vi "8HP_Standard_Clone.vi"(0 "Single 8HP":T1) -> (2 "DAQ Error":errorcluster, 3 "All samples out":sgl[][](array[numeric]), 4 "Ch No":i16[](array[numeric]), 5 "Index":i32[](array[numeric]), 6 "Sampling Rate Hz":dbl)   [LabVIEW 2021]
doc: "Use this plug-in with the Nathan 7609 data acquisition system"
uses:
  Device ID port info.ctl
  ctls/8HP_Cmd (USB).ctl
  Globals/Meas_global.vi
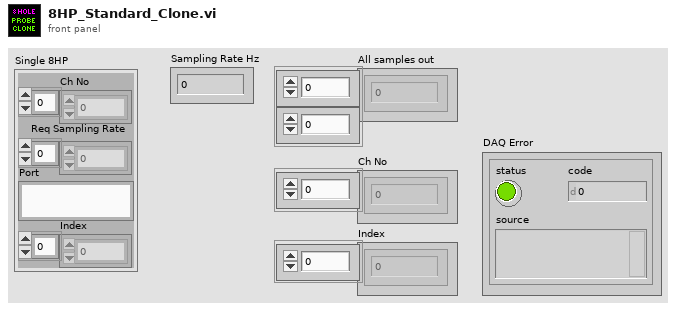
[diagram p1: front panel]
types:
  T1 = typedef "Device ID port info.ctl" = cluster{"Ch No":i16[], "Req Sampling Rate":dbl[], "Port":string, "Index":i32[]}
  T2 = typedef "8HP_Cmd (USB).ctl" = string
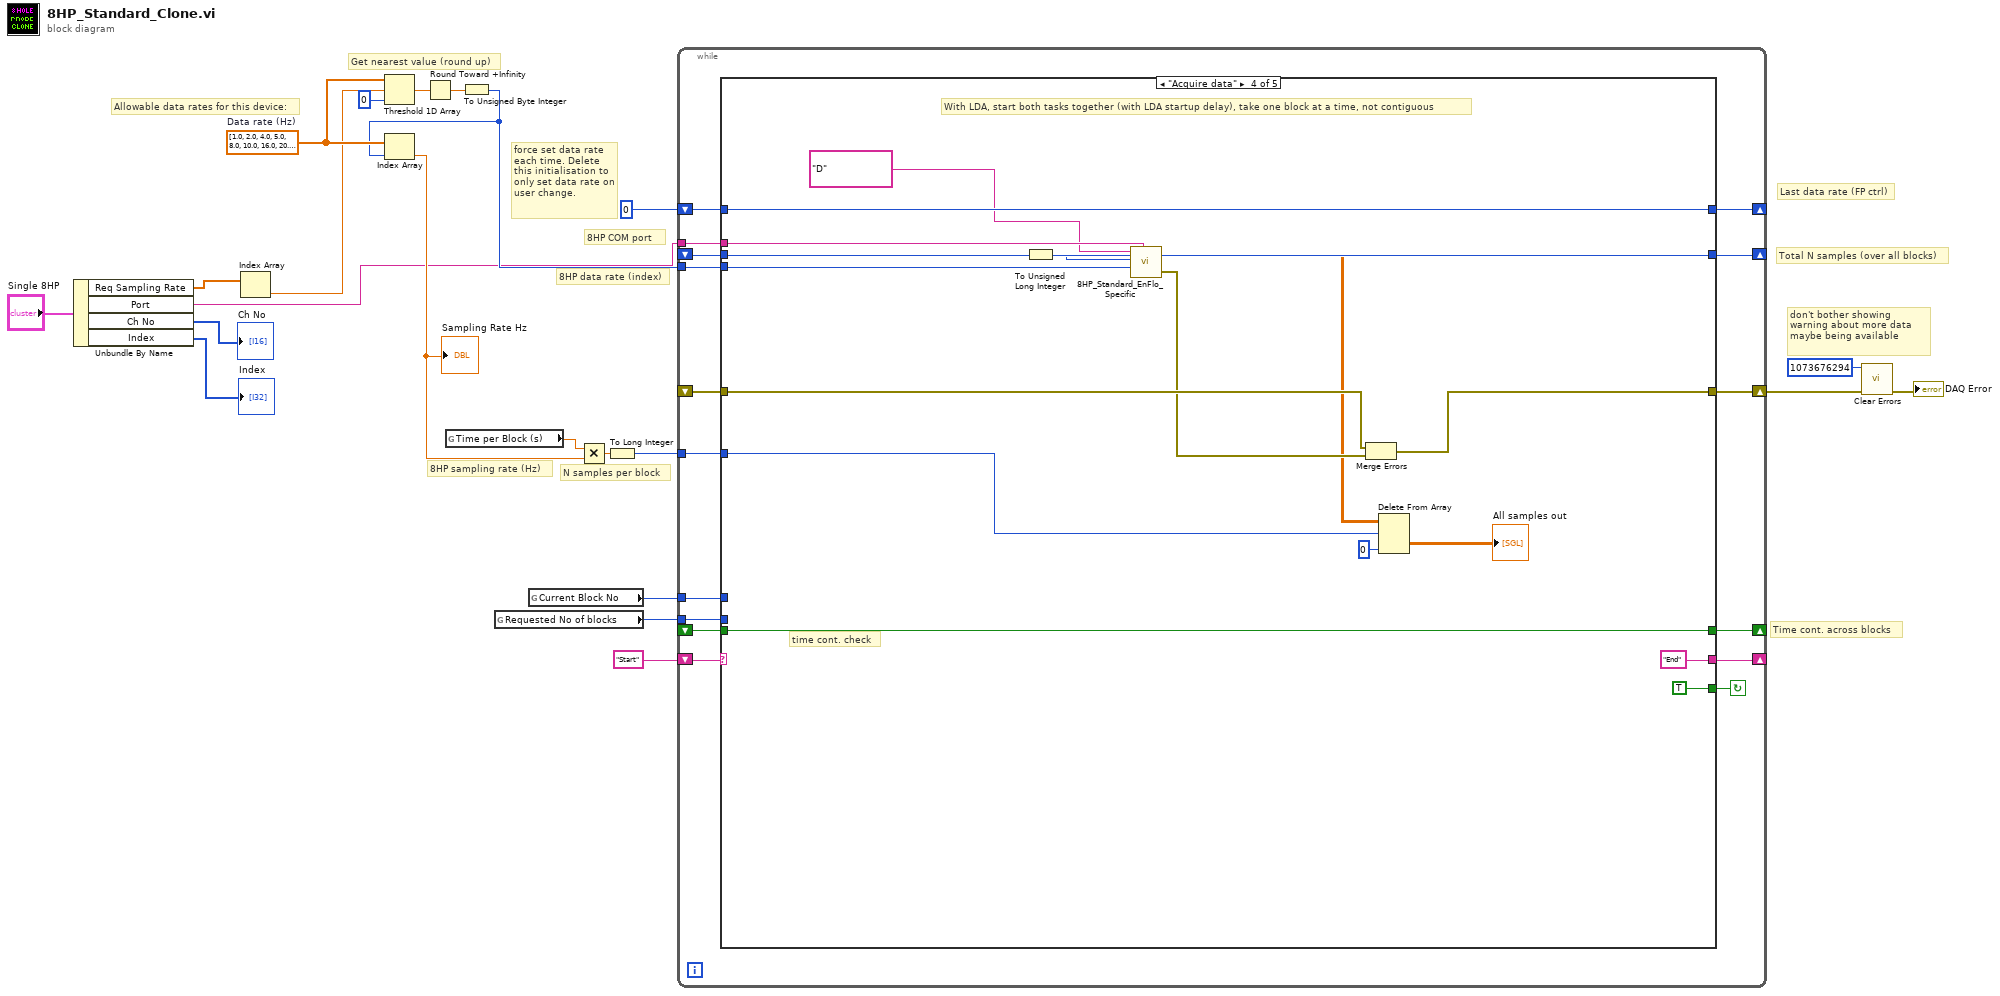
[diagram p0: block diagram]
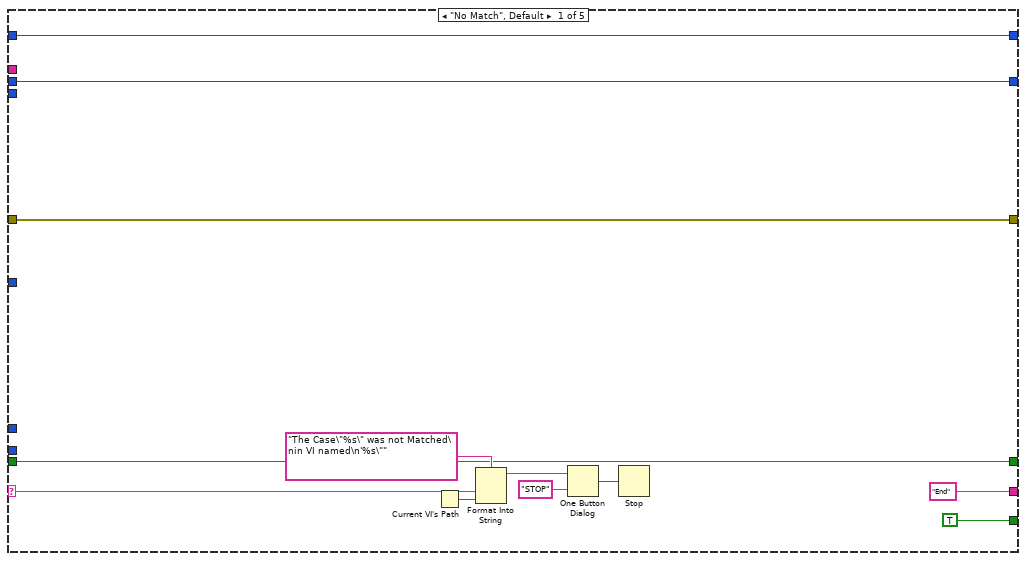
[diagram p2: hidden frame]
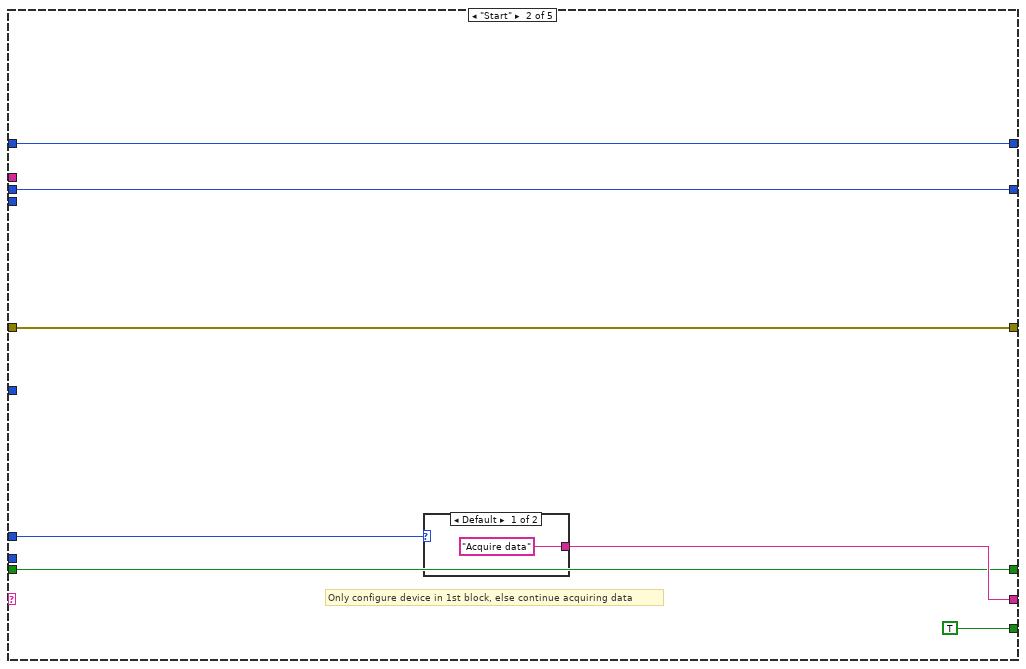
[diagram p3: hidden frame]
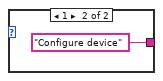
[diagram p4: hidden frame]
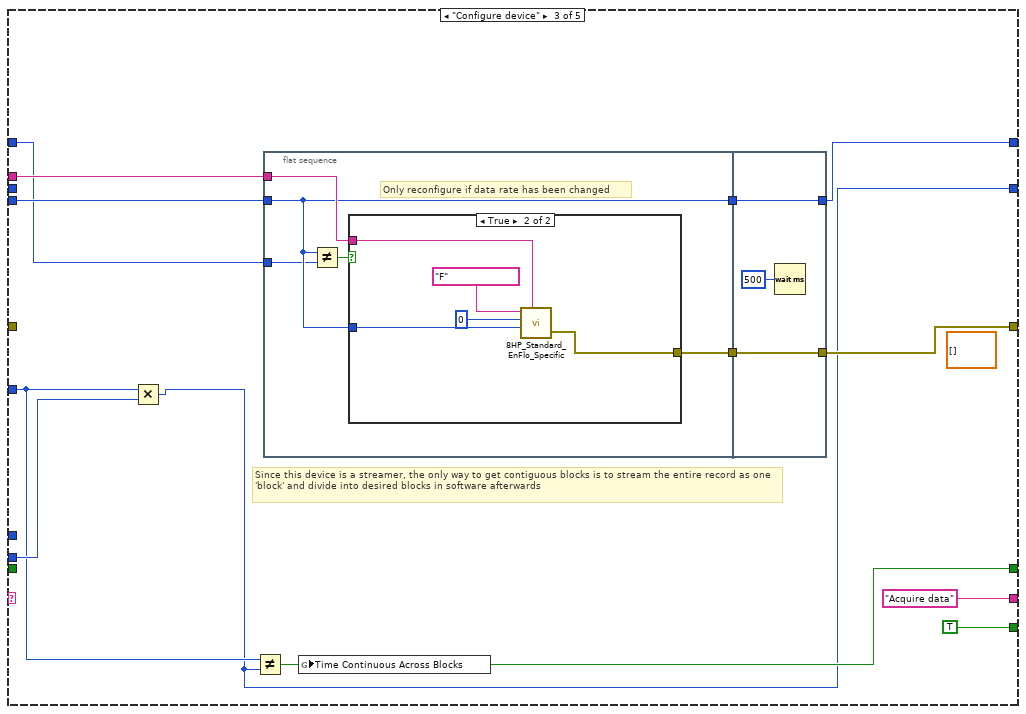
[diagram p5: hidden frame]
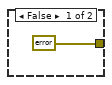
[diagram p6: hidden frame]
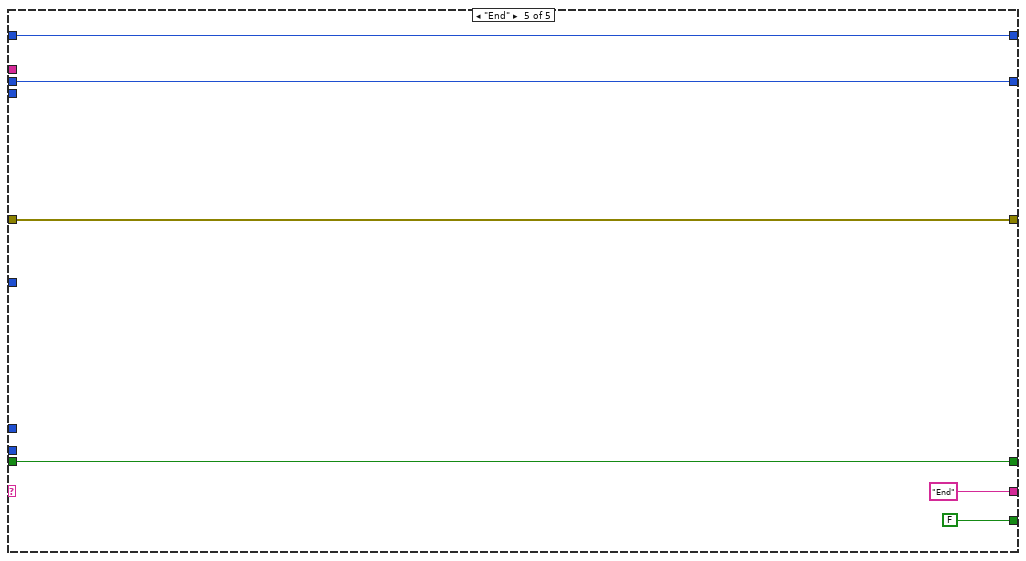
[diagram p7: hidden frame]
diagram:
  w13 = dbl[] [1.0, 2.0, 4.0, 5.0, 8.0, 10.0, 16.0, 20.0, 25.0, 32.0, 40.0, 50.0, 64.0, 80.0, 100.0, 125.0, 160.0, 200.0, 250.0, 320.0, 400.0, 500.0, 625.0, 800.0, 1000.0]  # Data rate (Hz)
  # "N samples per block"
  # "8HP sampling rate (Hz)"
  # "8HP COM port"
  # "8HP data rate (index)"
  # "Allowable data rates for this device:"
  # "Get nearest value (round up)"
  # "force set data rate each time. Delete this initialisation to only set data rate on user change."
  # "Last data rate (FP ctrl)"
  # "Total N samples (over all blocks)"
  # "don't bother showing warning about more data maybe being available"
  # "Time cont. across blocks"
  n1 = Unbundle By Name("Single 8HP") -> ("Req Sampling Rate"=w4:dbl[], "Port"=w5:string, "Ch No"=→"Ch No":i16[], "Index"=→"Index":i32[])
  n2 = Index Array(array=w4) -> (element=w3:dbl)  [unwired: 1 in]
  n3 = Threshold 1D Array(1:0 ("start index (0)"), 2:w3, 3:w13) -> (0:w14:dbl)
  n4 = Round Toward +Infinity(x=w14) -> (ceil(x): smallest int >= x=w12:dbl)
  n5 = global read "Meas_global.vi" "Time per Block (s)"() -> (w11:dbl)
  n6 = To Unsigned Byte Integer(number=w12) -> (unsigned 8bit integer=w7:u8)
  n7 = Index Array(array=w13, index=w7) -> (element=w8:dbl)
  "Sampling Rate Hz" <- w8
  n8 = global read "Meas_global.vi" "Requested No of blocks"() -> (w20:i32)
  n9 = global read "Meas_global.vi" "Current Block No"() -> (w21:i32)
  n10 = Multiply(x=w11, y=w8) -> (x*y=w10:dbl)
  n11 = To Long Integer(number=w10) -> (32bit integer=w9:i32)
  n12 = while {
    shift-left: "Start" -> [w38]
    shift-right: [w31] -> _
    tunnel: w9 -> [w37]
    tunnel: w21 -> [w36]
    tunnel: w20 -> [w34]
    shift-right: [w32] -> w17
    shift-left: _ -> [w33]
    shift-right: [w30] -> _
    shift-left: _ -> [w29]
    tunnel: w5 -> [w28]
    tunnel: w7 -> [w27]
    shift-right: [w26] -> _
    shift-left: _ -> [w25]
    shift-right: [w24] -> _
    shift-left: u8 0 ("Pressure data rate (Hz)") -> [w23]
    stop <- w35 continue-if-true
    n13 = case shown="\"Acquire data\"" w38 {
      selector: w38 -> [w43 _ _ _ _]
      tunnel: ["End" w54 "Acquire data" ("f") "End" "End" ("f")] -> w31
      tunnel: w37 -> [_ _ w68 w97 _]
      tunnel: w36 -> [_ w55 _ _ _]
      tunnel: [TRUE TRUE TRUE TRUE FALSE] -> w35
      tunnel: w34 -> [_ _ w71 _ _]
      tunnel: w33 -> [w42 w56 _ w100 w105]
      tunnel: [w42 w56 w70 w98 w105] -> w32
      tunnel: [w41 w53 w67 w99 w106] -> w30
      tunnel: w29 -> [w41 w53 _ w99 w106]
      tunnel: w28 -> [_ _ w66 w96 _]
      tunnel: w27 -> [_ _ w65 w95 _]
      tunnel: [w39 w51 w62 w93 w103] -> w26
      tunnel: w25 -> [w39 w51 _ w93 w103]
      tunnel: [w40 w52 w64 w94 w104] -> w24
      tunnel: w23 -> [w40 w52 w63 w94 w104]
      frame "No Match", Default {
        n14 = Current VI's Path() -> (path=w46:path)
        n15 = Format Into String(format string="The Case\"%s\" was not Matched\nin VI named\n'%s\"" ("Format String"), w43, w46) -> (resulting string=w49:string)  [unwired: 2 in, 1 out]
        n16 = One Button Dialog(message=w49, button name ("OK")="STOP") -> (true=w47:bool)
        n17 = Stop(stop? (T)=w47) -> ()
      }
      frame "Start" {
        # "Only configure device in 1st block, else continue acquiring data"
        n18 = case shown="Default" w55 {
          tunnel: ["Acquire data" ("f") "Configure device" ("f")] -> w54
          frame Default {
          }
          frame 1 {
          }
        }
      }
      frame "Configure device" {
        (unwired) sgl[][] [] ("Channel volts")
        # "Since this device is a streamer, the only way to get contiguous blocks is to stream the entire record as one 'block' and divide into desired blocks in software afterwards"
        n19 = Multiply(x=w68, y=w71) -> (x*y=w62:i32)
        n20 = Not Equal?(x=w68, y=w62) -> (x != y?=w67:bool)
        n21 = flat-sequence {
          tunnel: w66 -> [w76]
          tunnel: w65 -> [w74]
          tunnel: w63 -> [w73]
          tunnel: [w77] -> w61
          tunnel: [w74] -> w60
          tunnel: [w85] -> w64
          tunnel: [w86] -> w70
          tunnel: w61 -> [w86]
          tunnel: w60 -> [w85]
          frame #0 {
            # "Only reconfigure if data rate has been changed"
            n22 = Not Equal?(x=w74, y=w73) -> (x != y?=w75:bool)
            n23 = case shown="True" w75 {
              tunnel: [errorcluster {"status"=FALSE, "code"=0, "source"=""} ("error IO") w80] -> w77
              tunnel: w76 -> [_ w79]
              tunnel: w74 -> [_ w81]
              frame False {
              }
              frame True {
                n24 = call "8HP_Standard_EnFlo_Specific.vi"("COM port"=w79, "Set data rate (Hz)"=w81, "N samples"=u32 0, "Command"=T2 "F") -> ("Error"=w80:errorcluster)  [unwired: 2 in, 1 out]
              }
            }
          }
          frame #1 {
            n25 = Wait (ms)(milliseconds to wait=u32 500) -> ()  [unwired: 1 out]
          }
        }
        n26 = global write "Meas_global.vi" "Time Continuous Across Blocks"(w67) -> ()
      }
      frame "Acquire data" {
        # "time cont. check"
        # "With LDA, start both tasks together (with LDA startup delay), take one block at a time, not contiguous"
        n27 = To Unsigned Long Integer(number=w93) -> (unsigned 32bit integer=w87:u32)
        n28 = call "8HP_Standard_EnFlo_Specific.vi"("COM port"=w96, "Set data rate (Hz)"=w95, "N samples"=w87, "Command"=T2 "D") -> ("Error"=w90:errorcluster, "All samples out"=w89:sgl[][])  [unwired: 2 in]
        n29 = Merge Errors(w100, w90) -> (w98:errorcluster)
        n30 = Delete From Array(array=w89, length=w97, index (col)=0 ("disabled index (col)")) -> (deleted portion=→"All samples out":sgl[][])  [unwired: 1 in, 1 out]
      }
      frame "End" {
      }
    }
  }
  n31 = call <vilib>:"Clear Errors.vi"("error in (no error)"=w17, "specific error code to clear (0: all)"=1073676294) -> ("error out"=→"DAQ Error":errorcluster)  [unwired: 4 in, 1 out]
